vi "Find All Uses.IPE Unbundle.vi"(9 "Fully Qualified Array":string[](array[string]), 10 "dotted name":cluster{"dotted name":string[]}, 11 "VIs":refnum<vi>[](array[refnum])) -> (3 "results":refnum<vi>[](array[refnum]))   [LabVIEW 2020]
uses:
  <vilib>/Utility/traverseref.llb/TRef TravTarget.ctl
  <vilib>/Utility/traverseref.llb/VI Scripting - Traverse.lvlib
  <vilib>/Utility/Data Type/NI_Data Type.lvlib
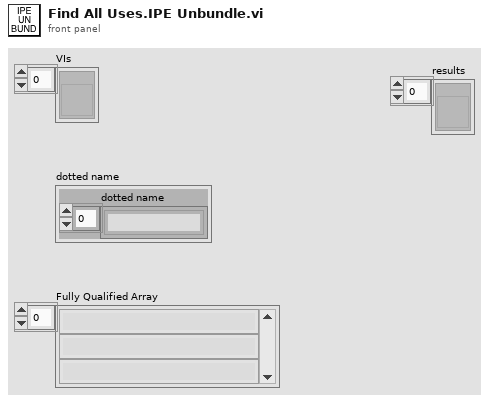
[diagram p1: front panel]
types:
  T1 = typedef "TRef TravTarget.ctl" = enum16{"FP", "BD", "Other"}
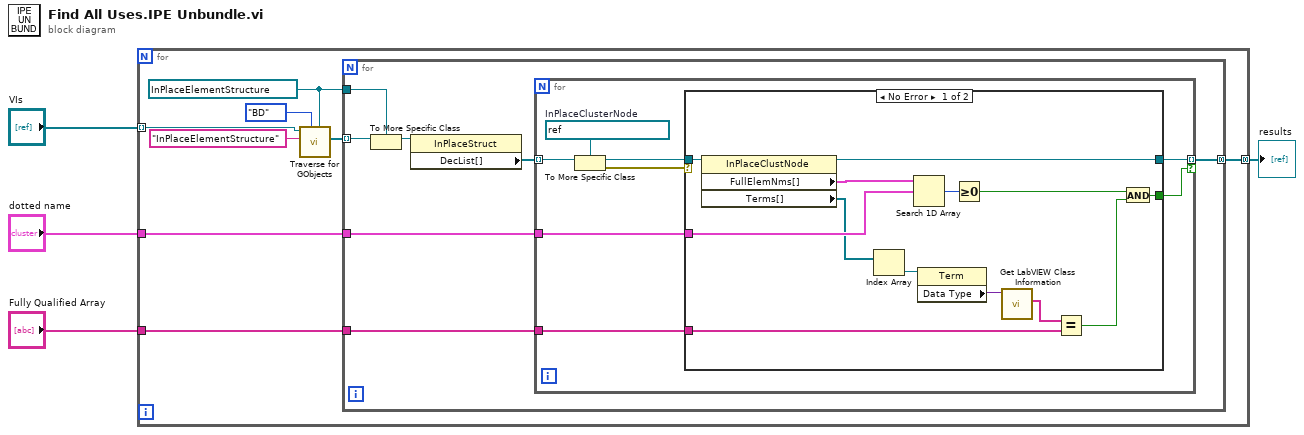
[diagram p0: block diagram]
diagram:
  n1 = for {
    tunnel: "VIs" -> [w12] mode=indexing
    tunnel: "dotted name" -> [w7]
    tunnel: [w6] -> w1 mode=concatenating
    tunnel: "Fully Qualified Array" -> [w5]
    w8 = refnum<vi> refnum ("Other Refnum")
    n2 = call <vilib>:"Traverse for GObjects.vi"("Other Refnum"=w8, "Traverse Target"=TRef_TravTarget."BD", "Class Name"="InPlaceElementStructure", "VI Refnum"=w12) -> ("References"=w9:refnum<vi>[])  [unwired: 4 in, 3 out]
    n3 = for {
      tunnel: w9 -> [w19] mode=indexing
      tunnel: w8 -> [w18]
      tunnel: w7 -> [w14]
      tunnel: [w13] -> w6 mode=concatenating
      tunnel: w5 -> [w16]
      n4 = To More Specific Class(target class=w18, reference=w19) -> (specific class reference=w17:refnum<vi>)  [unwired: 1 in, 1 out]
      n5 = property class="InPlaceStruct"(reference=w17) -> ("DecList[]"=w15:refnum<vi>[])  [unwired: 1 in, 2 out]
      n6 = for {
        tunnel: w16 -> [w27]
        tunnel: w15 -> [w26] mode=indexing
        tunnel: w14 -> [w22]
        tunnel: [w21] -> w13 mode=indexing if=w20
        w25 = refnum<vi> refnum  # InPlaceClusterNode
        n7 = To More Specific Class(target class=w25, reference=w26) -> (specific class reference=w23:refnum<vi>, error out=w24:errorcluster)  [unwired: 1 in]
        n8 = case shown="No Error" w24 {
          tunnel: w27 -> [w36 _]
          tunnel: [w33 _] -> w20
          tunnel: w23 -> [w32 _]
          tunnel: w22 -> [w30 _]
          tunnel: [w28 _] -> w21
          frame No Error {
            n9 = property class="InPlaceClustNode"(reference=w32) -> (reference out=w28:refnum<vi>, "FullElemNms[]"=w31:cluster{string[]}[], "Terms[]"=w29:refnum<vi>[])  [unwired: 1 in, 1 out]
            n10 = Index Array(array=w29) -> (element=w39:refnum<vi>)  [unwired: 1 in]
            n11 = Search 1D Array(1D array=w31, element=w30) -> (index of element=w40:i32)  [unwired: 1 in]
            n12 = property class="Term"(reference=w39) -> ("Data Type"=w38:variant)  [unwired: 1 in, 2 out]
            n13 = Greater Or Equal To 0?(x=w40) -> (x >= 0?=w34:bool)
            n14 = call <vilib>:"Get LabVIEW Class Information.vi"("variant"=w38) -> ("qualified LabVIEW class name"=w37:string[])  [unwired: 8 in, 2 out]
            n15 = Equal?(x=w37, y=w36) -> (x = y?=w35:bool)
            n16 = And(x=w34, y=w35) -> (x .and. y?=w33:bool)
          }
          frame Error {
          }
        }
      }
    }
  }
  "results" <- w1
